vi "RT Driver VI.vi"(6 "Device Clock":string, 9 "Device Inputs FIFO":refnum<k33>, 10 "Device Outputs FIFO":refnum<k33>, 11 "Device Reference":T1 format="%.0x") -> ()   [LabVIEW 2019, in "RMXVisaControl Engine.lvlib"]
uses:
  RMXVisaControl Engine.lvlib
  <vilib>/NI VeriStand/Custom Device API/Custom Device Item Ref.ctl
  <vilib>/NI VeriStand/Custom Device API/Custom Device Channel Type.ctl
  <vilib>/NI VeriStand/Custom Device API/Message Response (String).ctl
  <vilib>/NI VeriStand/Custom Device API/Message Response (Byte Array).ctl
  Shared/Constants.vi
  <vilib>/NI VeriStand/Custom Device API/Get Item Property (String).vi
  <vilib>/NI VeriStand/Custom Device API/Get Item Property (I32).vi
  <vilib>/NI VeriStand/Custom Device API/Custom Device API.lvlib
  <vilib>/NI VeriStand/Custom Device Tools/Custom Device Utility Library/Custom Device Utility Library.lvlib
  Shared/RMXVisaControl Shared.lvlib
  <instrlib>/NI RMX-412x Power Supplies/NI RMX-412x Power Supplies.lvlib
panel:
  in  "Initialization Status Notifier":refnum<notifier>
  in  "Status Notifier":refnum<notifier>
  # "Custom Device Template\nv1.0"
  # "Use this template as a starting point for creating a custom device code module. The input controls shown here are specially named controls that the system will use to provide the device loop with data. The controls are not required for the device loop to run. For instance, if the device doesn't produce any output data, then you don't need the Device Outputs FIFO control. If you do use these controls, however, they need to have these exact names to be functional."
  # "The optional status notifier element is used to notify the RT engine of the last state of the custom device, and to indicate the device has completed execution. If this control is not used, a default No Error value is returned to the system when the device finishes execution.\n\nNote: This error state is not checked until the system shuts down. Use an output status channel to send more immediate status values to the system."
  # "This optional input can be used to send the VeriStand Engine the final status of the custom device initalization process. If this control exists on the custom device front panel, the VeriStand Engine will wait for a status update before starting up. If the custom device reports an error, that will abort the execution of the current configuration in the VeriStand Engine.\n\nThis control can be deleted if the custom device does not need to send the initialization status update."
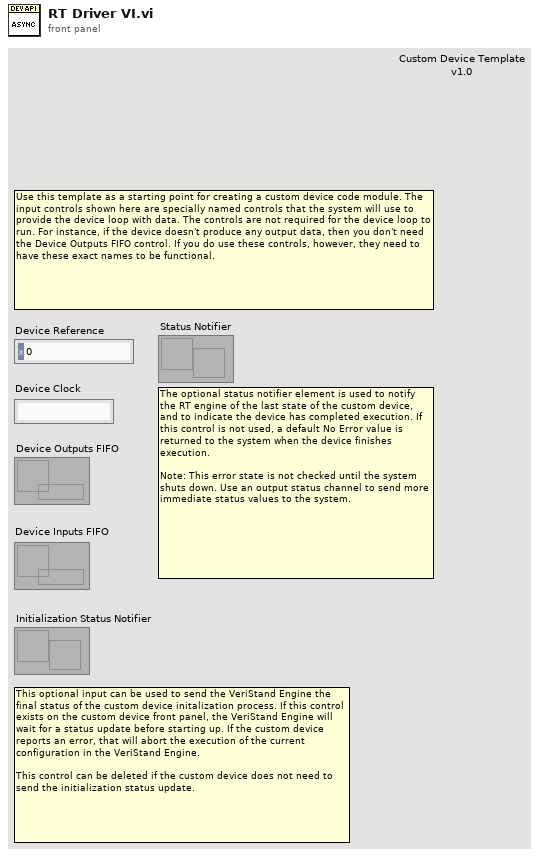
[diagram p1: front panel]
types:
  T1 = typedef "Custom Device API.lvlib/Custom Device Item Ref.ctl" = u64
  T2 = typedef "Custom Device API.lvlib/Custom Device Channel Type.ctl" = enum16{"Input", "Output"}
  T3 = typedef "Custom Device API.lvlib/Custom Device Engine Event Ref.ctl" = refnum<event-registration>
  T4 = typedef "Custom Device API.lvlib/Message Response (String).ctl" = cluster{"Response":string, "Error":errorcluster}
  T5 = typedef "Custom Device API.lvlib/Message Response (Byte Array).ctl" = cluster{"Response":u8[], "Error":errorcluster}
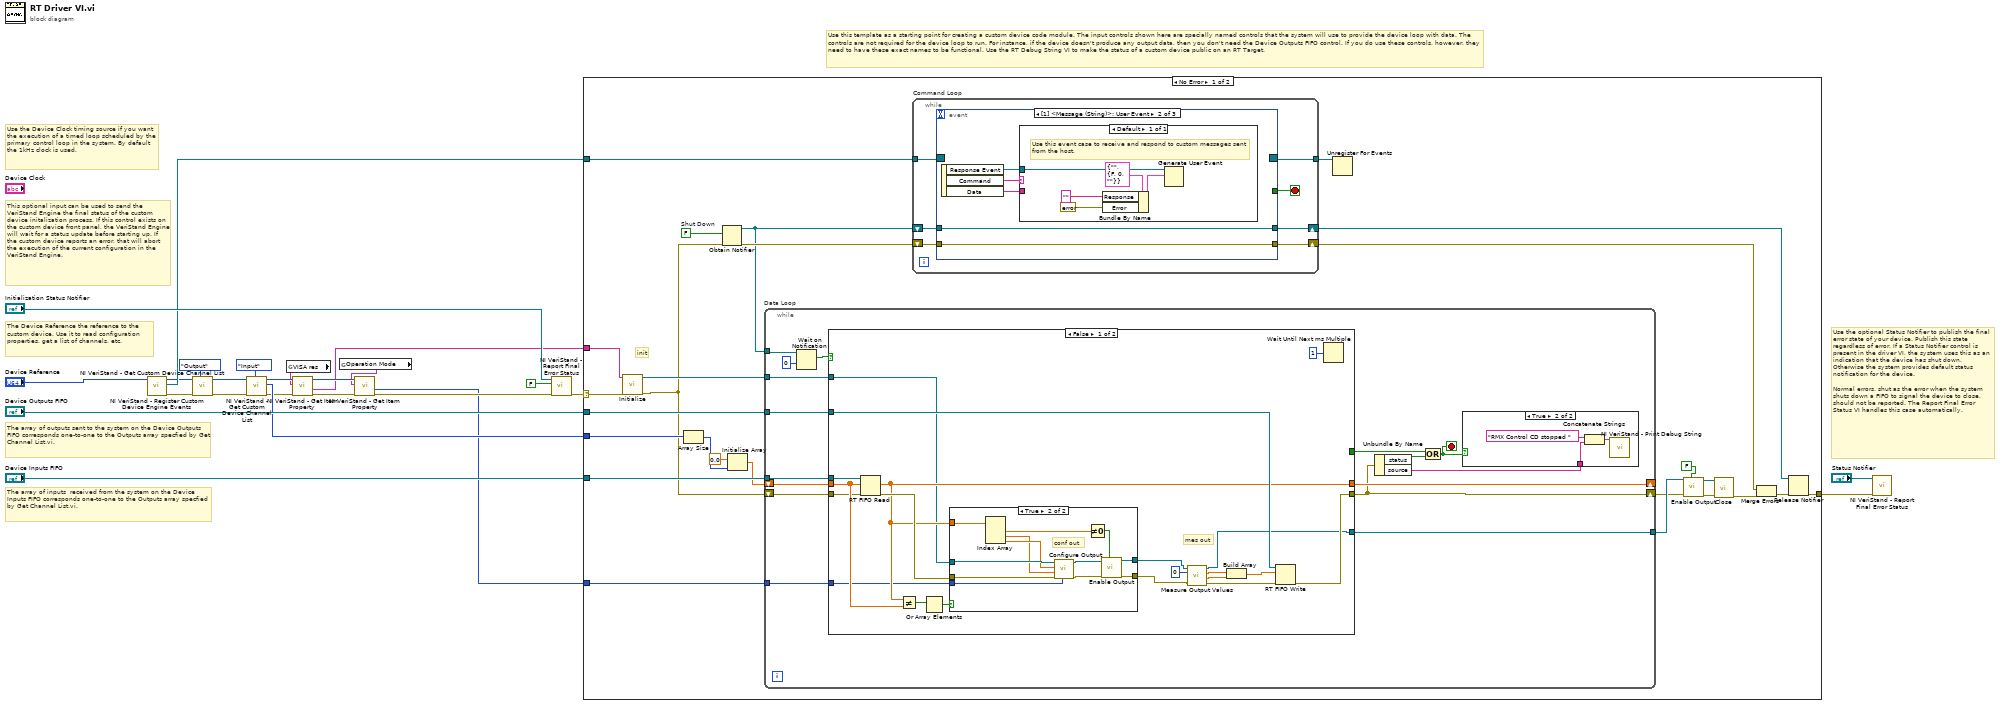
[diagram p0: block diagram]
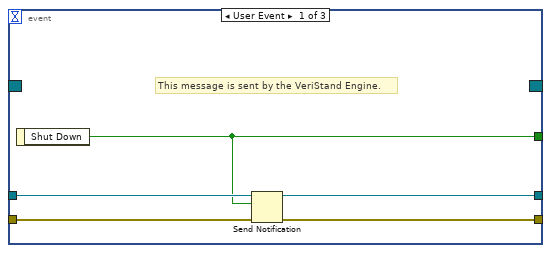
[diagram p2: hidden frame]
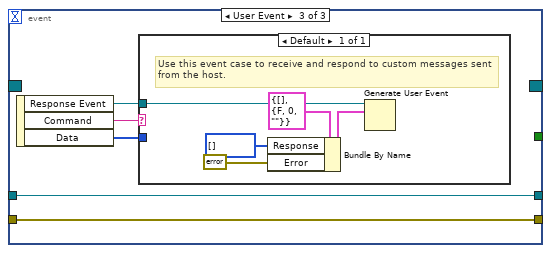
[diagram p3: hidden frame]
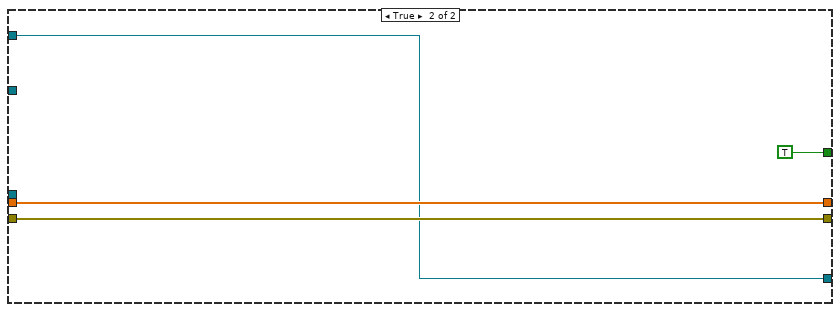
[diagram p6: hidden frame]
diagram:
  # "This optional input can be used to send the VeriStand Engine the final status of the custom device initalization process. If this control exists on the custom device front panel, the VeriStand Engine will wait for a status update before starting up. If the custom device reports an error, that will abort the execution of the current configuration in the VeriStand Engine."
  # "The array of inputs  received from the system on the Device Inputs FIFO corresponds one-to-one to the Outputs array specfied by Get Channel List.vi."
  # "Use the optional Status Notifier to publish the final error state of your device. Publish this state regardless of error. If a Status Notifier control is present in the driver VI, the system uses this as an indication that the device has shut down. Otherwise the system provides default status notification for the device.\n\nNormal errors, shut as the error when the system shuts down a FIFO to signal the device to close, should not be reported. The Report Final Error Status VI handles this case automatically."
  # "The array of outputs sent to the system on the Device Outputs FIFO corresponds one-to-one to the Outputs array specfied by Get Channel List.vi."
  # "The Device Reference the reference to the custom device. Use it to read configuration properties, get a list of channels, etc."
  # "Use the Device Clock timing source if you want the execution of a timed loop scheduled by the primary control loop in the system. By default the 1kHz clock is used."
  # "Use this template as a starting point for creating a custom device code module. The input controls shown here are specially named controls that the system will use to provide the device loop with data. The controls are not required for the device loop to run. For instance, if the device doesn't produce any output data, then you don't need the Device Outputs FIFO control. If you do use these controls, however, they need to have these exact names to be functional. Use the RT Debug String VI to make the status of a custom device public on an RT Target."
  n1 = call <vilib>:"NI VeriStand - Register Custom Device Engine Events.vi"("Device Ref in"="Device Reference") -> ("error out"=w25:errorcluster, "Custom Device Engine Event Ref"=w15:T3, "Device Ref out"=w12:T1)  [unwired: 8 in]
  n2 = call <vilib>:"NI VeriStand - Get Custom Device Channel List.vi"("Channel Type"=Custom_Device_Channel_Type."Output", "error in (no error)"=w25, "Device Ref in"=w12) -> ("error out"=w19:errorcluster, "Device Ref out"=w20:T1)  [unwired: 7 out]
  n3 = call <vilib>:"NI VeriStand - Get Custom Device Channel List.vi"("Channel Type"=Custom_Device_Channel_Type."Input", "error in (no error)"=w19, "Device Ref in"=w20) -> ("error out"=w9:errorcluster, "Specified Channel Ref List"=w17:T1[], "Device Ref out"=w8:T1)  [unwired: 6 out]
  n4 = global read "Constants.vi" "VISA res"() -> (w7:string)
  n5 = call-poly <vilib>:"NI VeriStand - Get Item Property.vi"("error in (no error)"=w9, "Property Name"=w7, "Item Ref in"=w8) -> ("error out"=w4:errorcluster, "Value"=w2:string, "Item Ref out"=w6:T1)  [unwired: 5 in, 1 out]
  n6 = global read "Constants.vi" "Operation Mode"() -> (w5:string)
  n7 = call-poly <vilib>:"NI VeriStand - Get Item Property.vi"("error in (no error)"=w4, "Property Name"=w5, "Item Ref in"=w6) -> ("error out"=w3:errorcluster, "Value"=w1:i32)  [unwired: 5 in, 2 out]
  n8 = call <vilib>:"NI VeriStand - Report Final Error Status.vi"("error in (no error)"=w3, "Filter FIFO & Shutdown Errors (T)"=FALSE ("Filter FIFO Errors (T)"), "Status Notifier"="Initialization Status Notifier") -> ("error out"=w11:errorcluster)  [unwired: 8 out]
  n9 = case shown="No Error" w11 {
    selector: w11 -> [w33 w141]
    tunnel: "Device Outputs FIFO" -> [w50 _]
    tunnel: "Device Inputs FIFO" -> [w49 _]
    tunnel: w17 -> [w46 _]
    tunnel: w15 -> [w44 _]
    tunnel: [w42 w141] -> w14
    tunnel: w2 -> [w32 _]
    tunnel: w1 -> [w36 _]
    frame No Error {
      w43 = FALSE  # Shut Down
      # "init"
      n10 = call <instrlib>:"Initialize.vi"("error in (no error)"=w33, "VISA resource name"=w32) -> ("error out"=w34:errorcluster, "VISA resource name out"=w35:refnum<visa-resource-name>)  [unwired: 8 in]
      n11 = Array Size(array=w46) -> (size(s)=w45:i32)
      n12 = Obtain Notifier(notification data type=w43, error in (no error)=w34) -> (notifier out=w40:refnum<notifier>, error out=w51:errorcluster)  [unwired: 2 in, 1 out]
      n13 = Initialize Array(0.0 ("element"), w45) -> (w47:dbl[])
      n14 = while "Data Loop" {
        shift-right: [w97] -> _
        shift-left: w47 -> [w98]
        shift-right: [w90] -> w29
        shift-left: w34 -> [w99]
        tunnel: w50 -> [w96]
        tunnel: w49 -> [w95]
        tunnel: w40 -> [w93]
        tunnel: w35 -> [w87]
        tunnel: [w86] -> w30
        tunnel: w36 -> [w84]
        stop <- w85 stop-if-true
        n15 = Wait on Notification(notifier=w93, timeout in ms (-1)=0) -> (notification=w92:bool)  [unwired: 2 in, 3 out]
        n16 = case shown="False" w92 {
          tunnel: w99 -> [w115 w139]
          tunnel: w98 -> [w120 w140]
          tunnel: [w116 w140] -> w97
          tunnel: w96 -> [w122 _]
          tunnel: w95 -> [w121 _]
          tunnel: [w113 w139] -> w90
          tunnel: [_ TRUE] -> w91
          tunnel: w87 -> [w114 w137]
          tunnel: [w105 w137] -> w86
          tunnel: w84 -> [w110 _]
          frame False {
            # "mes out"
            n17 = RT FIFO Read(0:w121, 1:w120, 3:w115) -> (9:w116:dbl[], 11:w117:errorcluster)  [unwired: 4 out]
            n18 = Not Equal?(x=w116, y=w120) -> (x != y?=w119:bool[])
            n19 = Or Array Elements(Boolean array=w119) -> (logical OR=w118:bool)
            n20 = case shown="True" w118 {
              tunnel: w114 -> [w123 w129]
              tunnel: w117 -> [w124 w128]
              tunnel: [w124 w133] -> w107
              tunnel: w116 -> [_ w136]
              tunnel: [w123 w134] -> w108
              tunnel: w110 -> [_ w127]
              frame False {
              }
              frame True {
                # "conf out"
                n21 = Index Array(array=w136) -> (element #1=w135:dbl, element #2=w125:dbl, element #3=w126:dbl)  [unwired: 3 in]
                n22 = call <instrlib>:"Configure Output.vi"("Operation Mode (0: Constant Current)"=w127, "error in (no error)"=w128, "Output Voltage (0 V)"=w125, "Output Current (0 A)"=w126, "VISA resource name"=w129) -> ("error out"=w131:errorcluster, "VISA resource name out"=w132:refnum<visa-resource-name>)  [unwired: 5 in]
                n23 = Not Equal To 0?(x=w135) -> (x != 0?=w130:bool)
                n24 = call <instrlib>:"Enable Output.vi"("Enable Output (F: Disable)"=w130, "error in (no error)"=w131, "VISA resource name"=w132) -> ("error out"=w133:errorcluster, "VISA resource name out"=w134:refnum<visa-resource-name>)  [unwired: 7 in]
              }
            }
            n25 = call <instrlib>:"Measure Output Values.vi"("error in (no error)"=w107, "Wait Before Query (1550 ms)"=u32 0, "VISA resource name"=w108) -> ("error out"=w106:errorcluster, "Current Output"=w103:dbl, "Voltage Output"=w104:dbl, "VISA resource name out"=w105:refnum<visa-resource-name>)  [unwired: 5 in]
            n26 = Build Array(w104, w103) -> (w112:dbl[])
            n27 = RT FIFO Write(0:w122, 1:w112, 3:w106) -> (11:w113:errorcluster)  [unwired: 1 in, 4 out]
            n28 = Wait Until Next ms Multiple(millisecond multiple=u32 1 ("milliseconds to wait")) -> ()  [unwired: 1 out]
          }
          frame True {
          }
        }
        n29 = Unbundle By Name(w90) -> ("status"=w89:bool, "source"=w88:string)
        n30 = Compound Arithmetic op=OR(w91, w89) -> (w85:bool)
        n31 = case shown="True" w85 {
          tunnel: w88 -> [_ w100]
          frame False {
          }
          frame True {
            n32 = Concatenate Strings("RMX Control CD stopped " ("string"), w100) -> (w102:string)
            n33 = call <vilib>:"NI VeriStand - Print Debug String.vi"("Message"=w102) -> ()  [unwired: 10 in, 1 out]
          }
        }
      }
      n34 = while "Command Loop" {
        tunnel: w44 -> [w58]
        tunnel: [w57] -> w41
        shift-right: [w54] -> w39
        shift-left: w40 -> [w55]
        shift-right: [w52] -> w37
        shift-left: w51 -> [w53]
        stop <- w56 stop-if-true
        n35 = event shown="[1] <Message (String)>: User Event" {
          selector: w58 -> [_ _ _]
          dyn-events: [_ _ _] -> w57
          timeout: _ -> [_ _ _]
          tunnel: [w61 _ _] -> w56
          tunnel: w55 -> [w62 w66 w76]
          tunnel: [w63 w66 w76] -> w54
          tunnel: w53 -> [w60 w64 w74]
          tunnel: [w59 w64 w74] -> w52
          event User Event {
            # "This message is sent by the VeriStand Engine."
            n36 = event-data() -> ("Shut Down"=w61:bool)  [unwired: 1 in]
            n37 = Send Notification(notification=w61, notifier=w62, error in (no error)=w60) -> (notifier out=w63:refnum<notifier>, error out=w59:errorcluster)
          }
          event User Event {
            n38 = event-data() -> ("Response Event"=w65:refnum<user-event>, "Command"=w68:string, "Data"=w67:string)  [unwired: 1 in]
            n39 = case shown="Default" w68 {
              tunnel: w67 -> [_]
              tunnel: w65 -> [w73]
              frame Default {
                # "Use this event case to receive and respond to custom messages sent from the host."
                n40 = Bundle By Name(cluster=T4 {"Response"="", "Error"={"status"=FALSE, "code"=0, "source"=""}} ("event data"), "Response"="", "Error"=errorcluster {"status"=FALSE, "code"=0, "source"=""}) -> (w71:T4)
                n41 = Generate User Event(user event=w73, event data cluster=w71) -> ()  [unwired: 2 in, 2 out]
              }
            }
          }
          event User Event {
            n42 = event-data() -> ("Response Event"=w75:refnum<user-event>, "Command"=w78:string, "Data"=w77:u8[])  [unwired: 1 in]
            n43 = case shown="Default" w78 {
              tunnel: w77 -> [_]
              tunnel: w75 -> [w83]
              frame Default {
                # "Use this event case to receive and respond to custom messages sent from the host."
                n44 = Bundle By Name(cluster=T5 {"Response"=[], "Error"={"status"=FALSE, "code"=0, "source"=""}} ("event data"), "Response"=u8[] [], "Error"=errorcluster {"status"=FALSE, "code"=0, "source"=""}) -> (w80:T5)
                n45 = Generate User Event(user event=w83, event data cluster=w80) -> ()  [unwired: 2 in, 2 out]
              }
            }
          }
        }
      }
      n46 = Unregister For Events(event registration refnum=w41) -> ()  [unwired: 1 in, 1 out]
      n47 = call <instrlib>:"Enable Output.vi"("Enable Output (F: Disable)"=FALSE, "error in (no error)"=w29, "VISA resource name"=w30) -> ("error out"=w28:errorcluster, "VISA resource name out"=w27:refnum<visa-resource-name>)  [unwired: 7 in]
      n48 = call <instrlib>:"Close.vi"("error in (no error)"=w28, "VISA resource name"=w27) -> ("error out"=w26:errorcluster)  [unwired: 9 in]
      n49 = Merge Errors(w37, w26) -> (w38:errorcluster)
      n50 = Release Notifier(notifier=w39, error in (no error)=w38) -> (error out=w42:errorcluster)  [unwired: 1 in, 2 out]
    }
    frame Error {
    }
  }
  n51 = call <vilib>:"NI VeriStand - Report Final Error Status.vi"("error in (no error)"=w14, "Status Notifier"="Status Notifier") -> ()  [unwired: 1 in, 9 out]
